vi "kSACommDemoLauncher.vi"() -> ()   [LabVIEW 2019]
panel:
  in  "OK Button":bool
  in  "Connect":bool
  in  "IP Address":string="localhost"
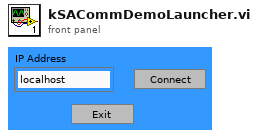
[diagram p1: front panel]
types:
  T1 = enum32{"Invalid", "Standard", "Closed", "Hidden", "Minimized", "Maximized"}
  T2 = enum32{"invalid app kind", "Development System", "Run Time System", "Student Edition", "Embedded LabVIEW", "Evaluation", "Custom"}
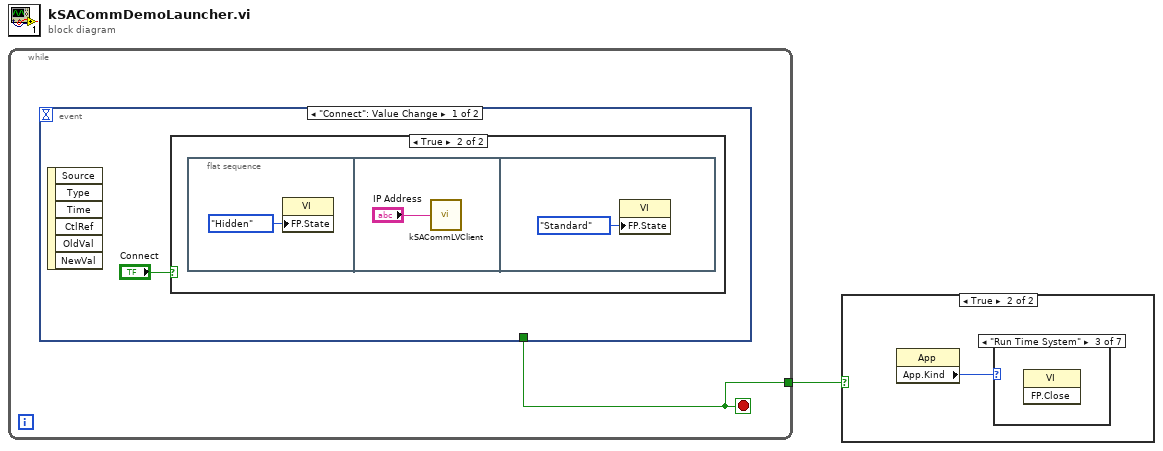
[diagram p0: block diagram]
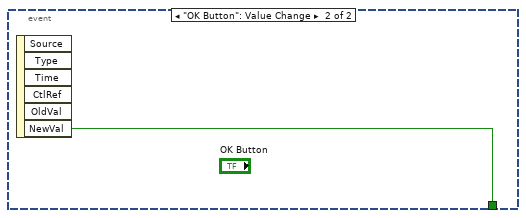
[diagram p10: hidden frame]
diagram:
  n1 = while {
    tunnel: [w2] -> w1
    stop <- w2 stop-if-true
    n2 = event shown="[0] \"Connect\": Value Change" {
      selector: _ -> [_ _]
      dyn-events: _ -> [_ _]
      timeout: _ -> [_ _]
      tunnel: [_ w7] -> w2
      event "Connect": Value Change {
        n3 = event-data() -> ()  [unwired: 1 in, 6 out]
        n4 = case shown="True" "Connect" {
          frame False {
          }
          frame True {
            n5 = flat-sequence {
              frame #0 {
                n6 = property class="VI"("FP.State"=T1."Hidden" ("Front Panel Window:State")) -> ()  [unwired: 2 in, 2 out]
              }
              frame #1 {
                n7 = call "kSACommLVClient.vi"("IP Address"="IP Address") -> ()  [unwired: 1 in]
              }
              frame #2 {
                n8 = property class="VI"("FP.State"=T1."Standard" ("Front Panel Window:State")) -> ()  [unwired: 2 in, 2 out]
              }
            }
          }
        }
      }
      event "OK Button": Value Change {
        n9 = event-data() -> ("NewVal"=w7:bool)  [unwired: 1 in, 5 out]
      }
    }
  }
  n10 = case shown="True" w1 {
    frame False {
    }
    frame True {
      n11 = property class="App"() -> ("App.Kind"=w8:T2)  [unwired: 2 in, 2 out]
      n12 = case shown="\"Run Time System\"" w8 {
        frame "invalid app kind", Default {
        }
        frame "Development System" {
        }
        frame "Run Time System" {
          n13 = invoke class="VI" method="FP.Close"() -> ()  [unwired: 3 in, 3 out]
        }
        frame "Student Edition" {
        }
        frame "Embedded LabVIEW" {
        }
        frame "Evaluation" {
        }
        frame "Custom" {
        }
      }
    }
  }
